vi "Read SEQ Frame.vi"(7 "error in (no error)":errorcluster, 8 "AOI List":i16[][](array[numeric]), 9 "Image Buffer In":T1, 10 "SEQ file refnum":refnum<file>) -> (0 "error out":errorcluster, 2 "Image Out":T1, 4 "Output frame height":i16, 5 "Output frame width":i16)   [LabVIEW 2016]
uses:
  <vilib>/vision/Image Controls.llb/IMAQ Image.ctl
  GLIMPSE Globals.vi
  <vilib>/vision/NI_Vision_Development_Module.lvlib
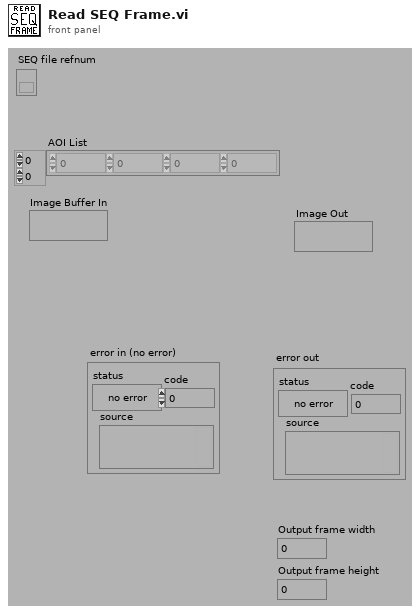
[diagram p1: front panel]
types:
  T1 = typedef "IMAQ Image.ctl" = refnum<image>
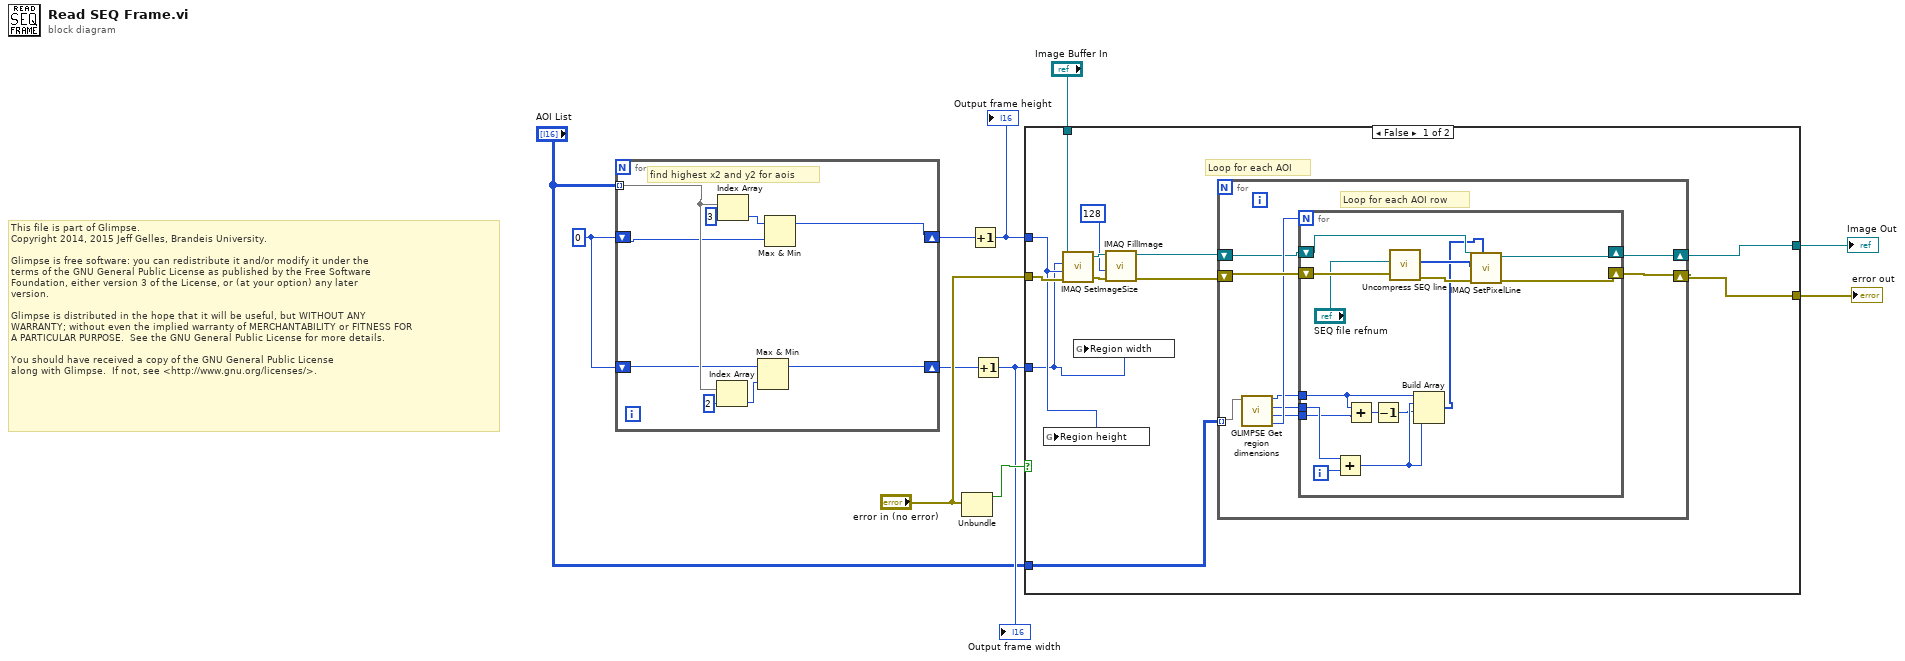
[diagram p0: block diagram]
diagram:
  w9 = i16 0
  # "This file is part of Glimpse. \nCopyright 2014, 2015 Jeff Gelles, Brandeis University.    \n\nGlimpse is free software: you can redistribute it and/or modify it under the \nterms of the GNU General Public License as published by the Free Software \nFoundation, either version 3 of the License, or (at your option) any later \nversion.\n\nGlimpse is distributed in the hope that it will be useful, but WITHOUT ANY \nWARRANTY; without even the implied warranty of MERCHANTABILITY or FITNESS FOR \nA PARTICULAR PURPOSE.  See the GNU General Public License for more details.\n\nYou should have received a copy of the GNU General Public License\nalong with Glimpse.  If not, see <http://www.gnu.org/licenses/>."
  n1 = for {
    tunnel: "AOI List" -> [w18] mode=indexing
    shift-right: [w15] -> w7
    shift-left: w9 -> [w12]
    shift-right: [w14] -> w8
    shift-left: w9 -> [w13]
    # "find highest x2 and y2 for aois"
    n2 = Index Array(array=w18, index=2) -> (element=w16:i16)
    n3 = Index Array(array=w18, index=3) -> (element=w17:i16)
    n4 = Max & Min(x=w13, y=w16) -> (max(x,y)=w14:i16)  [unwired: 1 out]
    n5 = Max & Min(x=w17, y=w12) -> (max(x,y)=w15:i16)  [unwired: 1 out]
  }
  n6 = Unbundle("error in (no error)") -> ("status"=w11:bool)  [unwired: 2 out]
  n7 = Increment(x=w7) -> (x+1=w6:i16)
  "Output frame height" <- w6
  n8 = Increment(x=w8) -> (x+1=w5:i16)
  "Output frame width" <- w5
  n9 = case shown="False" w11 {
    tunnel: "AOI List" -> [w32 _]
    tunnel: "error in (no error)" -> [w31 w57]
    tunnel: w5 -> [w29 _]
    tunnel: w6 -> [w30 _]
    tunnel: "Image Buffer In" -> [w25 w58]
    tunnel: [w22 w57] -> w2
    tunnel: [w21 w58] -> w1
    frame False {
      # "Loop for each AOI"
      n10 = global write "GLIMPSE Globals.vi" "Region height"(w30) -> ()
      n11 = call "IMAQ SetImageSize"("error in (no error)"=w31, "Y Resolution"=w30, "X Resolution"=w29, "Image"=w25) -> ("error out"=w28:errorcluster, "Image Out"=w27:T1)  [unwired: 1 out]
      n12 = global write "GLIMPSE Globals.vi" "Region width"(w29) -> ()
      n13 = call "IMAQ FillImage"("error in (no error)"=w28, "Pixel Value (U8, U16, I16, Float)"=u8 128, "Image"=w27) -> ("error out"=w24:errorcluster, "Image Out"=w23:T1)  [unwired: 4 in, 3 out]
      n14 = for {
        tunnel: w32 -> [w38] mode=indexing
        shift-right: [w40] -> w22
        shift-left: w24 -> [w41]
        shift-right: [w36] -> w21
        shift-left: w23 -> [w37]
        # "Loop for each AOI row"
        n15 = call "GLIMPSE Get region dimensions.vi"("x1y1x2y2"=w38) -> ("y size"=w39:u16, "x size"=w33:u16, "y origin"=w34:u16, "x origin"=w35:u16)  [unwired: 7 out]
        n16 = for {
          N: w39 -> [_]
          shift-right: [w53] -> w40
          shift-left: w41 -> [w56]
          shift-right: [w51] -> w36
          shift-left: w37 -> [w52]
          tunnel: w35 -> [w43]
          tunnel: w34 -> [w48]
          tunnel: w33 -> [w44]
          i -> [w49]
          n17 = Add(x=w48, y=w49) -> (x+y=w47:i32)
          n18 = Add(x=w43, y=w44) -> (x+y=w45:u16)
          n19 = Decrement(x=w45) -> (x-1=w46:u16)
          n20 = call "Uncompress SEQ line.vi"("error in"=w56, "SEQ file refnum"="SEQ file refnum") -> ("error out"=w54:errorcluster, "Pixel Array"=w50:u8[])  [unwired: 4 out]
          n21 = Build Array(w43, w47, w46, w47) -> (w42:i32[])
          n22 = call "IMAQ SetPixelLine"("Line Coordinates"=w42, "error in (no error)"=w54, "Pixels Line (U8)"=w50, "Image"=w52) -> ("error out"=w53:errorcluster, "Image Out"=w51:T1)  [unwired: 3 in, 3 out]
        }
      }
    }
    frame True {
    }
  }
  "error out" <- w2
  "Image Out" <- w1
